vi "Encoder Reading.vi"(3 "Position Reset":bool, 4 "Values":T1, 5 "Encoder Intputs":T3) -> (0 "output cluster":T1, 1 "Speed Output":T2, 2 "Position Output":T4)   [LabVIEW 2013]
uses:
  <vilib>/rvi/eio/common/nirviEmuTemplateMethod_errors.vi
  <vilib>/eio/EIONode/EIONode.xnode
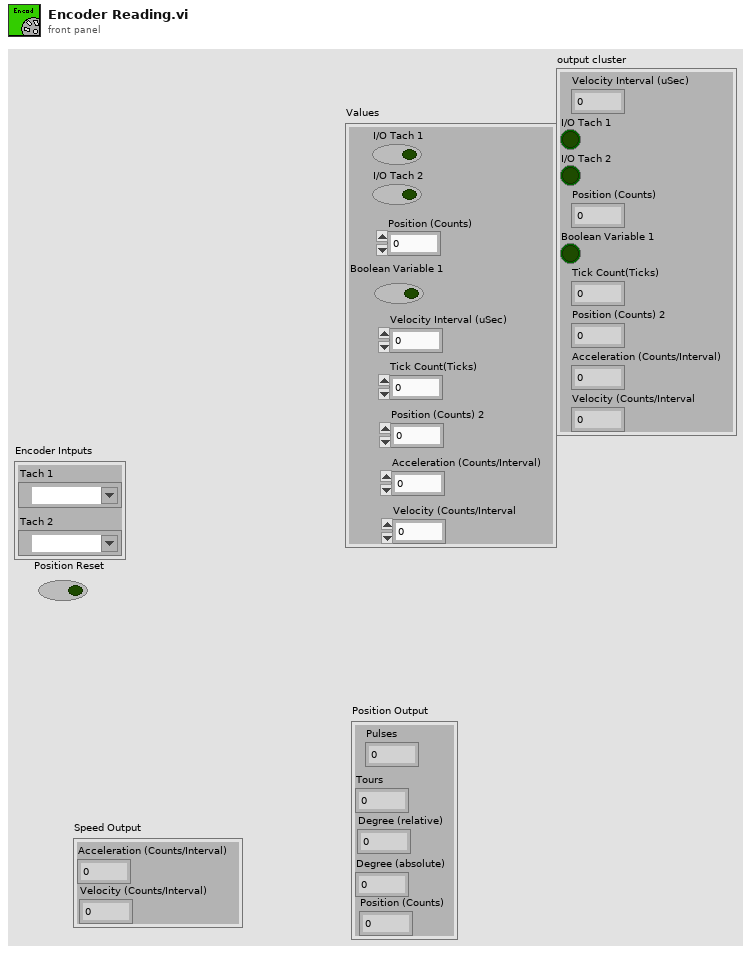
[diagram p1: front panel]
types:
  T1 = cluster{"Velocity Interval (uSec)":i32, "I/O Tach 1":bool, "I/O Tach 2":bool, "Position (Counts)":i16, "Boolean Variable 1":bool, "Tick Count(Ticks)":u32, "Position (Counts) 2":i16, "Acceleration (Counts/Interval)":i16, "Velocity (Counts/Interval":i16}
  T2 = cluster{"Velocity (Counts/Interval)":i32, "Acceleration (Counts/Interval)":i32}
  T3 = cluster{"Tach 2":refnum<k21>, "Tach 1":refnum<k21>}
  T4 = cluster{"Pulses":i32, "Degree (absolute)":i32, "Degree (relative)":i32, "Tours":i32, "Position (Counts)":i32}
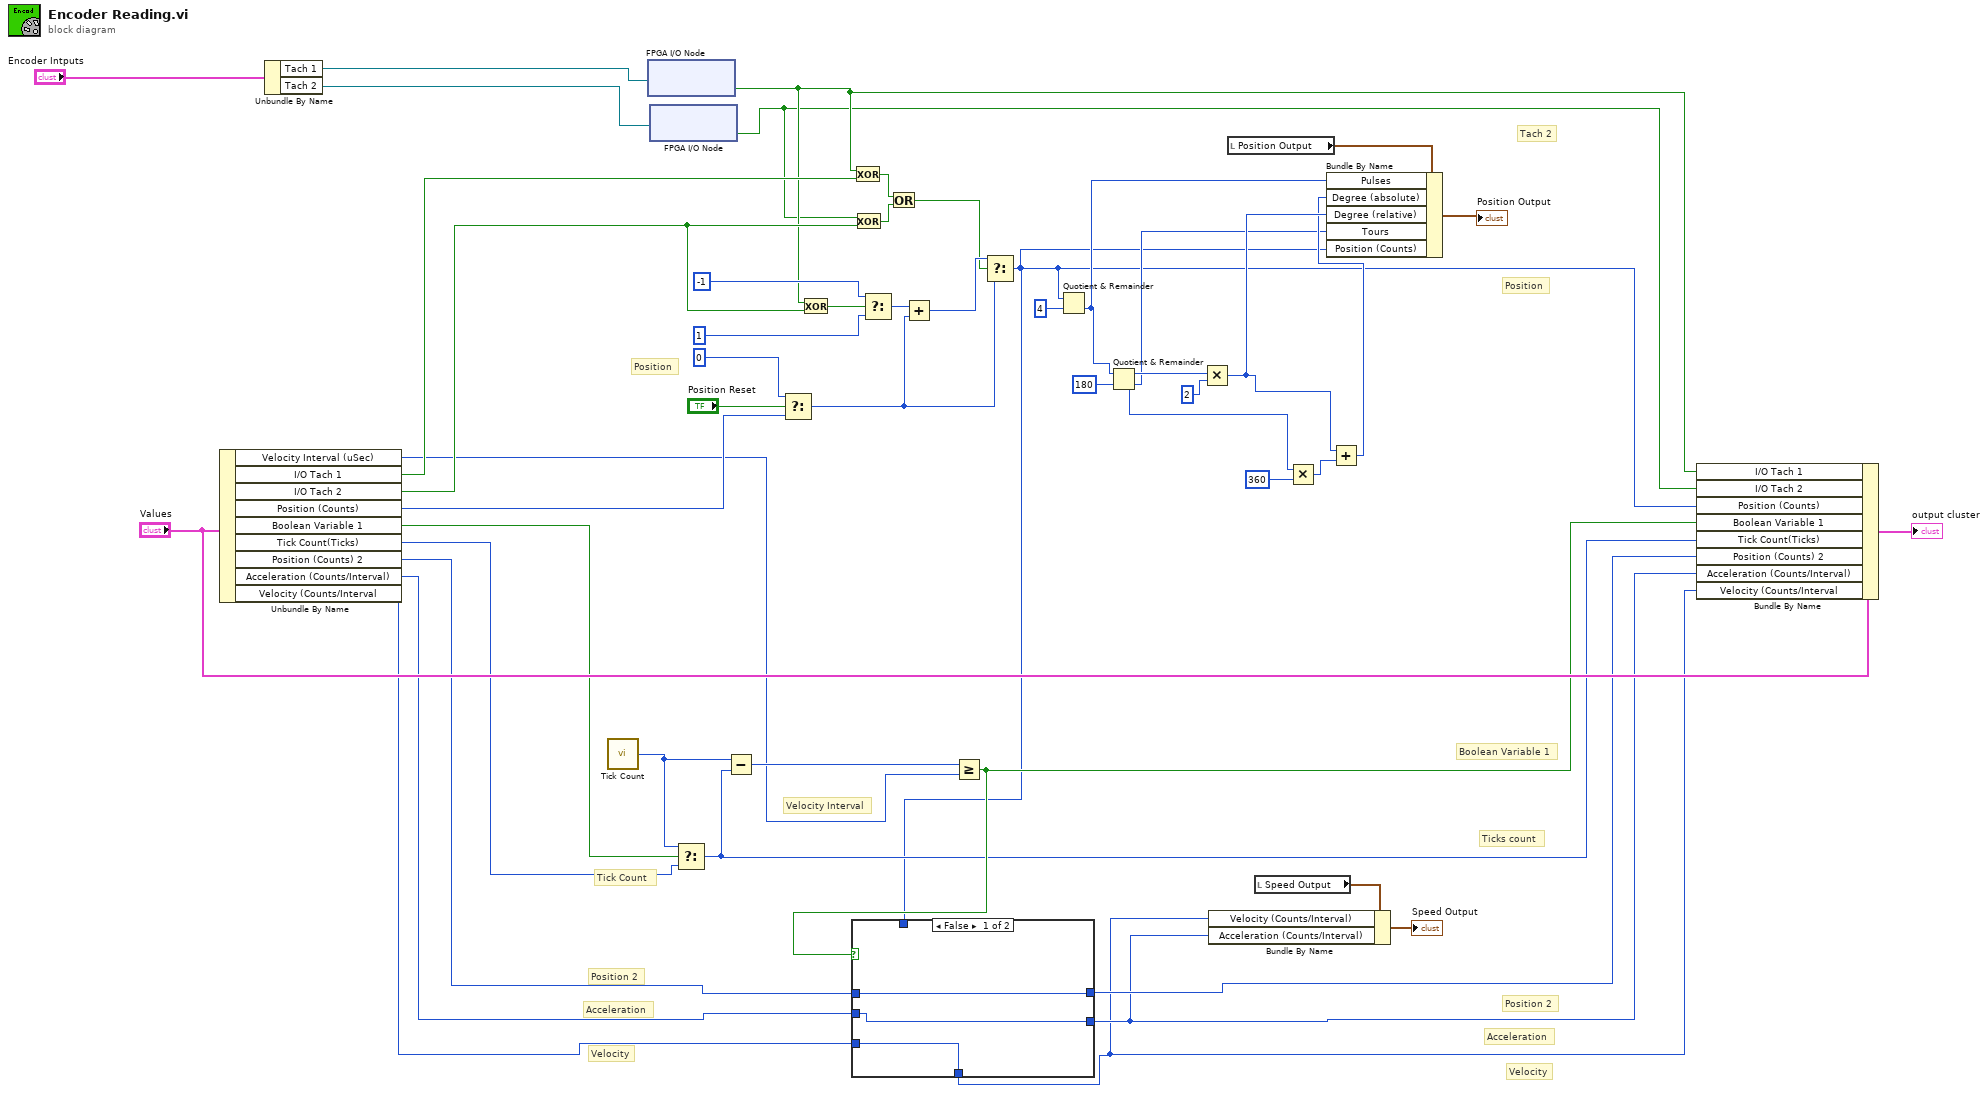
[diagram p0: block diagram]
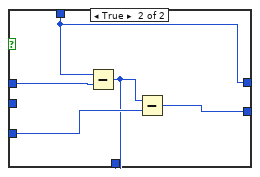
[diagram p2: hidden frame]
diagram:
  # "Position"
  # "Velocity Interval"
  # "Tick Count"
  # "Position 2"
  # "Acceleration"
  # "Velocity"
  # "Tach 2"
  # "Position"
  # "Boolean Variable 1"
  # "Ticks count"
  # "Position 2"
  # "Acceleration"
  # "Velocity"
  n1 = Unbundle By Name("Values") -> ("Velocity Interval (uSec)"=w16:i32, "I/O Tach 1"=w20:bool, "I/O Tach 2"=w19:bool, "Position (Counts)"=w18:i16, "Boolean Variable 1"=w17:bool, "Tick Count(Ticks)"=w15:u32, "Position (Counts) 2"=w12:i16, "Acceleration (Counts/Interval)"=w13:i16, "Velocity (Counts/Interval"=w14:i16)
  n2 = Unbundle By Name("Encoder Intputs") -> ("Tach 1"=w3:refnum<k21>, "Tach 2"=w2:refnum<k21>)
  n3 = call "Tick Count"() -> ("Tick Count(Ticks)"=w38:u32)
  n4 = xnode "FPGA I/O Node"("FPGA I/O In"=w3) -> ("I/O Item"=w11:bool)  [unwired: 1 out]
  n5 = xnode "FPGA I/O Node"("FPGA I/O In"=w2) -> ("I/O Item"=w10:bool)  [unwired: 1 out]
  n6 = Select(t=w38, s=w17, f=w15) -> (s? t:f=w8:u32)
  n7 = Subtract(x=w38, y=w8) -> (x-y=w39:u32)
  n8 = Select(t=i16 0, s="Position Reset", f=w18) -> (s? t:f=w40:i16)
  n9 = Exclusive Or(1:w19, 2:w11) -> (0:w37:bool)
  n10 = Exclusive Or(1:w20, 2:w11) -> (0:w47:bool)
  n11 = Exclusive Or(1:w19, 2:w10) -> (0:w46:bool)
  n12 = Select(t=i16 -1, s=w37, f=i16 1) -> (s? t:f=w42:i16)
  n13 = Or(x=w47, y=w46) -> (x .or. y?=w35:bool)
  n14 = Add(x=w42, y=w40) -> (x+y=w41:i16)
  n15 = Greater Or Equal?(x=w39, y=w16) -> (x >= y?=w9:bool)
  n16 = Select(t=w41, s=w35, f=w40) -> (s? t:f=w4:i16)
  n17 = case shown="False" w9 {
    tunnel: w12 -> [w52 w57]
    tunnel: w4 -> [_ w56]
    tunnel: [w52 w56] -> w7
    tunnel: [w51 w55] -> w6
    tunnel: w14 -> [w50 w54]
    tunnel: [w50 w53] -> w5
    tunnel: w13 -> [w51 _]
    frame False {
    }
    frame True {
      n18 = Subtract(x=w56, y=w57) -> (x-y=w53:i16)
      n19 = Subtract(x=w53, y=w54) -> (x-y=w55:i16)
    }
  }
  n20 = Quotient & Remainder(x=w4, y=i16 4) -> (floor(x/y)=w28:i16)  [unwired: 1 out]
  n21 = Quotient & Remainder(x=w28, y=i16 180) -> (x-y*floor(x/y)=w33:i16, floor(x/y)=w25:i16)
  n22 = Multiply(x=w33, y=i16 2) -> (x*y=w27:i16)
  n23 = local read "Position Output"() -> (w23:T4)
  n24 = local read "Speed Output"() -> (w22:T2)
  n25 = Bundle By Name(cluster=w22, "Velocity (Counts/Interval)"=w5, "Acceleration (Counts/Interval)"=w6) -> (→"Speed Output":T2)
  n26 = Multiply(x=w25, y=i16 360) -> (x*y=w30:i16)
  n27 = Add(x=w27, y=w30) -> (x+y=w26:i16)
  n28 = Bundle By Name(cluster=w23, "Pulses"=w28, "Degree (absolute)"=w26, "Degree (relative)"=w27, "Tours"=w25, "Position (Counts)"=w4) -> (→"Position Output":T4)
  n29 = Bundle By Name(cluster="Values", "I/O Tach 1"=w11, "I/O Tach 2"=w10, "Position (Counts)"=w4, "Boolean Variable 1"=w9, "Tick Count(Ticks)"=w8, "Position (Counts) 2"=w7, "Acceleration (Counts/Interval)"=w6, "Velocity (Counts/Interval"=w5) -> (→"output cluster":T1)
